vi "_set.vi"(2 "错误输入（无错误）":errorcluster, 3 "写入缓冲区":string, 4 "VISA资源名称输出 2":refnum<visa-resource-name>) -> (0 "错误输出":errorcluster, 1 "VISA资源名称输出":refnum<visa-resource-name>)   [LabVIEW 2017]
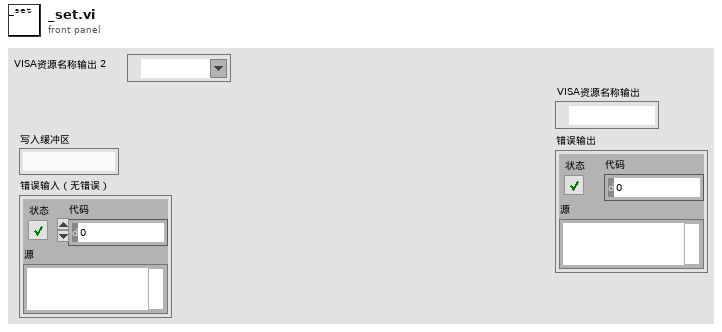
[diagram p1: front panel]
types:
  T1 = typedef "Semaphore RefNum" = refnum<k1>
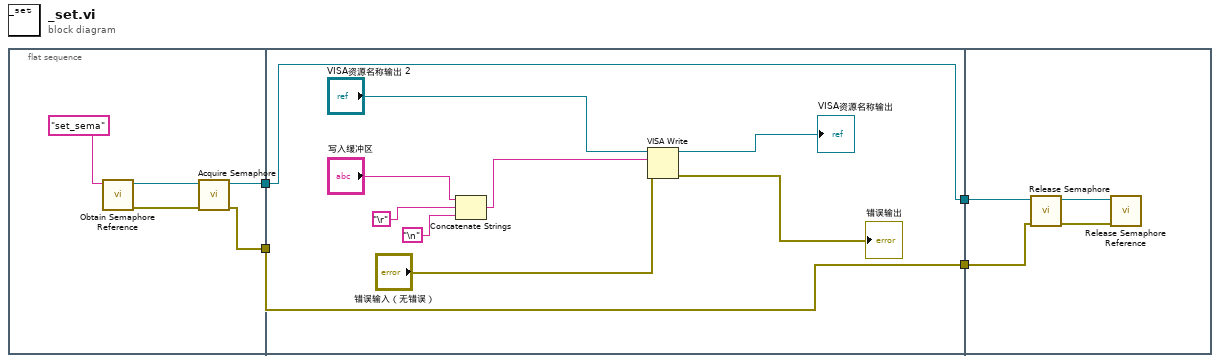
[diagram p0: block diagram]
diagram:
  n1 = flat-sequence {
    tunnel: [w6] -> w3
    tunnel: [w5] -> w1
    tunnel: [w11] -> w4
    tunnel: w3 -> [w11]
    tunnel: [w10] -> w2
    tunnel: w1 -> [w10]
    tunnel: w4 -> [w21]
    tunnel: w2 -> [w20]
    frame #0 {
      n2 = call <vilib>:"Obtain Semaphore Reference.vi"("name (unnamed)"="set_sema") -> ("error out"=w9:errorcluster, "semaphore"=w7:T1)  [unwired: 4 in, 1 out]
      n3 = call <vilib>:"Acquire Semaphore.vi"("error in (no error)"=w9, "semaphore"=w7) -> ("error out"=w5:errorcluster, "semaphore out"=w6:T1)  [unwired: 3 in, 1 out]
    }
    frame #1 {
      n4 = Concatenate Strings("写入缓冲区", "\r", "\n") -> (w15:string)
      n5 = VISA Write(VISA resource name="VISA资源名称输出 2", write buffer=w15, error in (no error)="错误输入（无错误）") -> (VISA resource name out=→"VISA资源名称输出":refnum<visa-resource-name>, error out=→"错误输出":errorcluster)  [unwired: 1 out]
    }
    frame #2 {
      n6 = call <vilib>:"Release Semaphore.vi"("error in (no error)"=w20, "semaphore"=w21) -> ("error out"=w22:errorcluster, "semaphore out"=w23:T1)  [unwired: 4 in]
      n7 = call <vilib>:"Release Semaphore Reference.vi"("error in (no error)"=w22, "semaphore"=w23) -> ()  [unwired: 8 in, 2 out]
    }
  }
